vi "Error Process.vi"(8 "error in (no error)":errorcluster, 11 "View Model":T1) -> (0 "error out":errorcluster)   [LabVIEW 2017]
doc: "Process provide centralized error handler for Elevator controller."
uses:
  View Model/Controls/View Model.ctl
  View Model/Controls/Shared Model.ctl
  Controls/Error Model.ctl
  Controls/Error Data.ctl
  Controls/Error Level.ctl
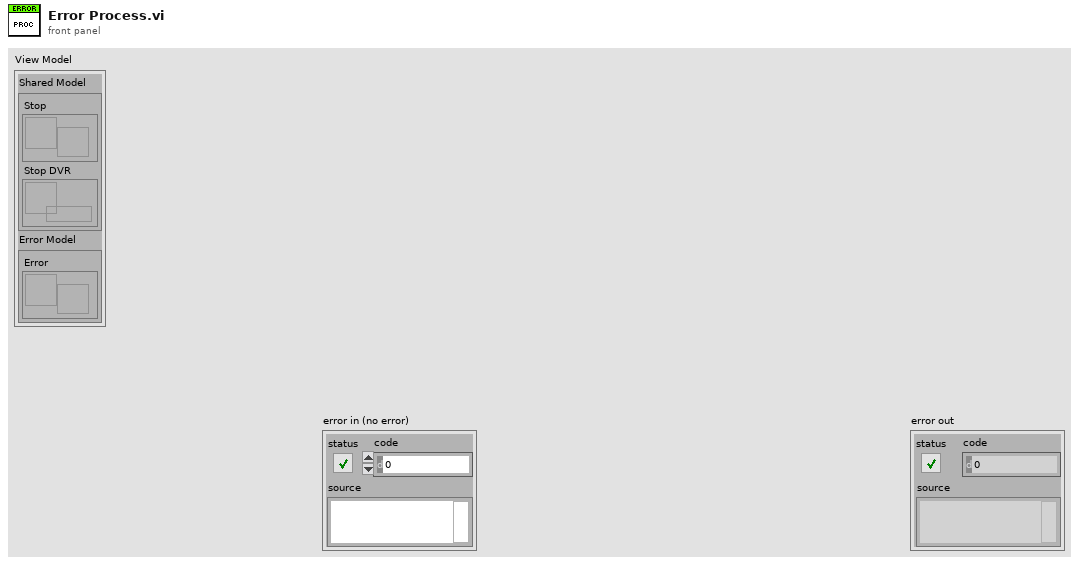
[diagram p1: front panel]
types:
  T1 = typedef "View Model.ctl" = cluster{"Shared Model":T2, "Error Model":T3}
  T2 = typedef "Shared Model.ctl" = cluster{"Stop":refnum<user-event>, "Stop DVR":refnum<data-value>}
  T3 = typedef "Error Model.ctl" = cluster{"Error":refnum<user-event>}
  T4 = typedef "Error Level.ctl" = enum16{"Console Error", "Sensor Interface IO Error", "Process Step Error"}
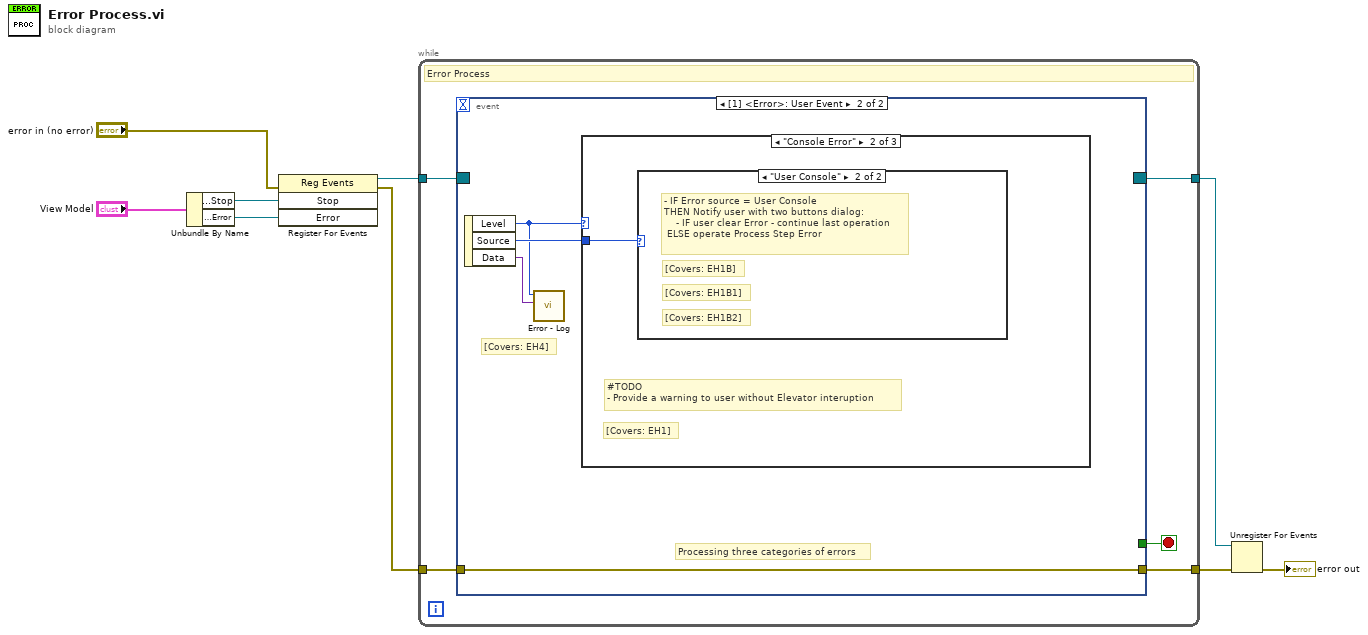
[diagram p0: block diagram]
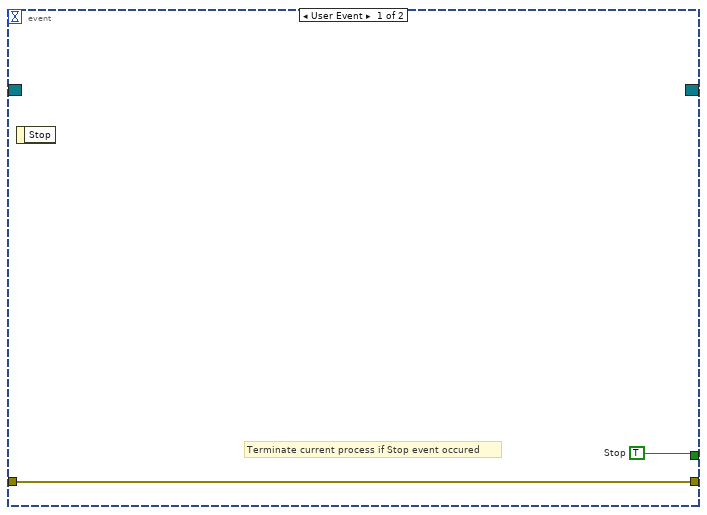
[diagram p2: hidden frame]
diagram:
  n1 = Unbundle By Name("View Model") -> ("Shared Model.Stop"=w9:refnum<user-event>, "Error Model.Error"=w1:refnum<user-event>)
  n2 = register-events(error in="error in (no error)", w9, w1) -> (reference out=w8:refnum<event-registration>, error out=w6:errorcluster)  [unwired: 1 in]
  n3 = while {
    tunnel: w8 -> [w14]
    tunnel: w6 -> [w13]
    tunnel: [w12] -> w3
    tunnel: [w10] -> w4
    stop <- w11 stop-if-true
    # "Error Process"
    n4 = event shown="[1] <Error>: User Event" {
      selector: w14 -> [_ _]
      dyn-events: [_ _] -> w10
      timeout: _ -> [_ _]
      tunnel: w13 -> [w16 w20]
      tunnel: [w16 w20] -> w12
      tunnel: [w15 _] -> w11
      event User Event {
        w15 = TRUE  # Stop
        # "Terminate current process if Stop event occured"
        n5 = event-data() -> ()  [unwired: 1 in, 1 out]
      }
      event User Event {
        # "[Covers: EH4]"
        # "Processing three categories of errors"
        n6 = event-data() -> ("Level"=w18:T4, "Source"=w19:enum16{"Display Console", "User Console"}, "Data"=w17:variant)  [unwired: 1 in]
        n7 = call "Error - Log.vi"("Data"=w17, "Level"=w18) -> ()  [unwired: 9 in, 1 out]
        n8 = case shown="\"Console Error\"" w18 {
          tunnel: w19 -> [_ w21 _]
          frame Default {
            # "for additional errors"
          }
          frame "Console Error" {
            # "[Covers: EH1]"
            # "#TODO\n- Provide a warning to user without Elevator interuption"
            n9 = case shown="\"User Console\"" w21 {
              frame "Display Console", Default {
                # "[Covers: EH1A]"
                # "- IF Error source = Display Console \nTHEN Notify user, clear error, \ncontinue last operation."
              }
              frame "User Console" {
                # "[Covers: EH1B2]"
                # "[Covers: EH1B1]"
                # "[Covers: EH1B]"
                # "- IF Error source = User Console \nTHEN Notify user with two buttons dialog:\n    - IF user clear Error - continue last operation\n ELSE operate Process Step Error"
              }
            }
          }
          frame "Sensor Interface IO Error", "Process Step Error" {
            # "[Covers: EH2]"
            # "#TODO\nExecutes Termination process"
          }
        }
      }
    }
  }
  n10 = Unregister For Events(event registration refnum=w4, error in=w3) -> (error out=→"error out":errorcluster)
